vi "raster_scan_ground_shutter_new1.vi"() -> ()   [LabVIEW 2014] (continued)
  out "Spectra":cluster{"X":dbl, "Y":dbl}[](graph)=[{"X"=0.0, "Y"=0.9945769033962795}, {"X"=1.0, "Y"=0.9947742774918267}, {"X"=2.0, "Y"=0.9948669642938777}, {"X"=3.0, "Y"=0.9936503120864774}, {"X"=4.0, "Y"=0.99410258502573}, {"X"=5.0, "Y"=0.9940668724529786}, {"X"=6.0, "Y"=0.9937261199251147}, {"X"=7.0, "Y"=0.9931260471704962}, {"X"=8.0, "Y"=0.992983146361495}, {"X"=9.0, "Y"=0.9929502642830587}, {"X"=10.0, "Y"=0.993348571521516}, {"X"=11.0, "Y"=0.993598876753815}, {"X"=12.0, "Y"=0.9934939146853311}, {"X"=13.0, "Y"=0.994586396575504}, {"X"=14.0, "Y"=0.9948678392216669}, {"X"=15.0, "Y"=0.9949446767024206}, {"X"=16.0, "Y"=0.9954073186324625}, {"X"=17.0, "Y"=0.9946994697141236}, {"X"=18.0, "Y"=0.9944550521013112}, {"X"=19.0, "Y"=0.9944548626426379}, {"X"=20.0, "Y"=0.9935020518216698}, {"X"=21.0, "Y"=0.993658626270429}, {"X"=22.0, "Y"=0.9930985706701053}, {"X"=23.0, "Y"=0.9927409549288653}, {"X"=24.0, "Y"=0.9933271800562766}, {"X"=25.0, "Y"=0.9933239327867504}, {"X"=26.0, "Y"=0.9936027818310011}, {"X"=27.0, "Y"=0.9941736390892316}, {"X"=28.0, "Y"=0.9944683191284457}, {"X"=29.0, "Y"=0.9946912128001987}, {"X"=30.0, "Y"=0.9949701648247575}, {"X"=31.0, "Y"=0.9954933893926244}, {"X"=32.0, "Y"=0.9953930559005679}, {"X"=33.0, "Y"=0.9953512482962834}, {"X"=34.0, "Y"=0.9949945889014346}, {"X"=35.0, "Y"=0.9945846796005057}, {"X"=36.0, "Y"=0.9945806119423862}, {"X"=37.0, "Y"=0.9940680651637547}, {"X"=38.0, "Y"=0.9934632136375385}, {"X"=39.0, "Y"=0.9938541294612084}, {"X"=40.0, "Y"=0.9939211970775383}, {"X"=41.0, "Y"=0.9943574368554471}, {"X"=42.0, "Y"=0.9940101330545833}, {"X"=43.0, "Y"=0.9951367236173629}, {"X"=44.0, "Y"=0.9947572071731021}, {"X"=45.0, "Y"=0.9959756804722151}, {"X"=46.0, "Y"=0.9956182213866881}, {"X"=47.0, "Y"=0.9955081448310908}, {"X"=48.0, "Y"=0.995631614186444}, {"X"=49.0, "Y"=0.9956208296036213}, {"X"=50.0, "Y"=0.9962532896605993}, {"X"=51.0, "Y"=0.9962533556114832}, {"X"=52.0, "Y"=0.9958614347766488}, {"X"=53.0, "Y"=0.9957461636865907}, {"X"=54.0, "Y"=0.9956406167835943}, {"X"=55.0, "Y"=0.9956854770758357}, {"X"=56.0, "Y"=0.9956615767212665}, {"X"=57.0, "Y"=0.9956945496935939}, {"X"=58.0, "Y"=0.9962324646454884}, {"X"=59.0, "Y"=0.9964947407469643}, {"X"=60.0, "Y"=0.9970926126529994}, {"X"=61.0, "Y"=0.9968670550577037}, {"X"=62.0, "Y"=0.9970965802345466}, {"X"=63.0, "Y"=0.9972656492697479}, {"X"=64.0, "Y"=0.9968582713175153}, {"X"=65.0, "Y"=0.9970401597074343}, {"X"=66.0, "Y"=0.9970443003613348}, {"X"=67.0, "Y"=0.9973501158902985}, {"X"=68.0, "Y"=0.9981303427188236}, {"X"=69.0, "Y"=0.9977305631322807}, {"X"=70.0, "Y"=0.9977540022221576}, {"X"=71.0, "Y"=0.9979177515384777}, {"X"=72.0, "Y"=0.9977070175561394}, {"X"=73.0, "Y"=0.9982594221394903}, {"X"=74.0, "Y"=0.9980605550971688}, {"X"=75.0, "Y"=0.9978803843894963}, {"X"=76.0, "Y"=0.9980351530513635}, {"X"=77.0, "Y"=0.997851075793747}, {"X"=78.0, "Y"=0.9977894200446173}, {"X"=79.0, "Y"=0.9980636064837063}, {"X"=80.0, "Y"=0.9985695417684551}, {"X"=81.0, "Y"=0.9983812791956344}, {"X"=82.0, "Y"=0.998341559725945}, {"X"=83.0, "Y"=0.9986510426559164}, {"X"=84.0, "Y"=0.9991944690408153}, {"X"=85.0, "Y"=0.9995105354611745}, {"X"=86.0, "Y"=0.9991164177012709}, {"X"=87.0, "Y"=0.9995787032972646}, {"X"=88.0, "Y"=0.999454788017559}, {"X"=89.0, "Y"=0.999155685132651}, {"X"=90.0, "Y"=0.9987649485431911}, {"X"=91.0, "Y"=0.9986068010093291}, {"X"=92.0, "Y"=0.9976290609707013}, {"X"=93.0, "Y"=0.9981984662044825}, {"X"=94.0, "Y"=0.9977038350208027}, {"X"=95.0, "Y"=0.9979091185166017}, {"X"=96.0, "Y"=0.9984387389872107}, {"X"=97.0, "Y"=0.998465208764674}, {"X"=98.0, "Y"=0.9984988692668328}, {"X"=99.0, "Y"=0.9985777685951757}, {"X"=100.0, "Y"=0.9992981103342568}, {"X"=101.0, "Y"=0.9992176789240342}, {"X"=102.0, "Y"=0.9993160506202576}, {"X"=103.0, "Y"=0.9989016439374092}, {"X"=104.0, "Y"=0.998344902827914}, {"X"=105.0, "Y"=0.9982534949398687}, {"X"=106.0, "Y"=0.9981679578327937}, {"X"=107.0, "Y"=0.9971053281612066}, {"X"=108.0, "Y"=0.9971389132184889}, {"X"=109.0, "Y"=0.9963932015726795}, {"X"=110.0, "Y"=0.997024447798127}, {"X"=111.0, "Y"=0.9970324424009313}, {"X"=112.0, "Y"=0.9965660403857277}, {"X"=113.0, "Y"=0.9967183745842016}, {"X"=114.0, "Y"=0.9964512134239439}, {"X"=115.0, "Y"=0.9970165326649953}, {"X"=116.0, "Y"=0.9970951875378874}, {"X"=117.0, "Y"=0.9973005892418015}, {"X"=118.0, "Y"=0.9963413510352245}, {"X"=119.0, "Y"=0.9971948818360715}, {"X"=120.0, "Y"=0.9965308996775175}, {"X"=121.0, "Y"=0.9963267133794433}, {"X"=122.0, "Y"=0.9962490289924059}, {"X"=123.0, "Y"=0.99548039025524}, {"X"=124.0, "Y"=0.9948693730639996}, {"X"=125.0, "Y"=0.9944480660225795}, {"X"=126.0, "Y"=0.9946001681176279}, {"X"=127.0, "Y"=0.9943400299459262}, {"X"=128.0, "Y"=0.9946766752271496}, {"X"=129.0, "Y"=0.9950541253232607}, {"X"=130.0, "Y"=0.9945720808080813}, {"X"=131.0, "Y"=0.9948365747834916}, {"X"=132.0, "Y"=0.9950096816408889}, {"X"=133.0, "Y"=0.9949251864213772}, {"X"=134.0, "Y"=0.9940405960933386}, {"X"=135.0, "Y"=0.9938257461507851}, {"X"=136.0, "Y"=0.9944341634194976}, {"X"=137.0, "Y"=0.9940765135946166}, {"X"=138.0, "Y"=0.9932345009989546}, {"X"=139.0, "Y"=0.9928583382361931}, {"X"=140.0, "Y"=0.9926401294064278}, {"X"=141.0, "Y"=0.9929389318614823}, {"X"=142.0, "Y"=0.9927168132710366}, {"X"=143.0, "Y"=0.9926980851100657}, {"X"=144.0, "Y"=0.9920478801636552}, {"X"=145.0, "Y"=0.9925539606832021}, {"X"=146.0, "Y"=0.9928183067524887}, {"X"=147.0, "Y"=0.9926309997007406}, {"X"=148.0, "Y"=0.9917379549723951}, {"X"=149.0, "Y"=0.9923930264472043}, {"X"=150.0, "Y"=0.9918422229407143}, {"X"=151.0, "Y"=0.9914120672419391}, {"X"=152.0, "Y"=0.99163739825362}, {"X"=153.0, "Y"=0.9919110399406977}, {"X"=154.0, "Y"=0.9921509491520646}, {"X"=155.0, "Y"=0.9919826244448052}, {"X"=156.0, "Y"=0.9915638810734073}, {"X"=157.0, "Y"=0.9919883739976783}, {"X"=158.0, "Y"=0.9920186750240084}, {"X"=159.0, "Y"=0.9919484618380446}, {"X"=160.0, "Y"=0.9914327944146301}, {"X"=161.0, "Y"=0.9914833838660724}, {"X"=162.0, "Y"=0.9909328552617234}, {"X"=163.0, "Y"=0.99087425566013}, {"X"=164.0, "Y"=0.9896353008053395}, {"X"=165.0, "Y"=0.9901551379155719}, {"X"=166.0, "Y"=0.9892554727011702}, {"X"=167.0, "Y"=0.9900682622175773}, {"X"=168.0, "Y"=0.9897916508753934}, {"X"=169.0, "Y"=0.990067512842968}, {"X"=170.0, "Y"=0.9899459386432332}, {"X"=171.0, "Y"=0.9911563889695773}, {"X"=172.0, "Y"=0.9906125677236967}, {"X"=173.0, "Y"=0.9911465853056776}, {"X"=174.0, "Y"=0.9909635003778303}, {"X"=175.0, "Y"=0.9904879603894554}, {"X"=176.0, "Y"=0.9906311459060286}, {"X"=177.0, "Y"=0.9901740860080628}, {"X"=178.0, "Y"=0.9897736777248581}, {"X"=179.0, "Y"=0.9891083590917772}, {"X"=180.0, "Y"=0.9885407356391681}, {"X"=181.0, "Y"=0.9887437574853996}, {"X"=182.0, "Y"=0.9875871706582002}, {"X"=183.0, "Y"=0.9884301915828902}, {"X"=184.0, "Y"=0.9880786140088792}, {"X"=185.0, "Y"=0.9888277232763419}, {"X"=186.0, "Y"=0.9890520421386713}, {"X"=187.0, "Y"=0.9895665359857829}, {"X"=188.0, "Y"=0.9899055459783636}, {"X"=189.0, "Y"=0.9904301218378724}, {"X"=190.0, "Y"=0.9902234343017942}, {"X"=191.0, "Y"=0.9901724736185524}, {"X"=192.0, "Y"=0.9901434464237711}, {"X"=193.0, "Y"=0.9895637959186443}, {"X"=194.0, "Y"=0.988702010117804}, {"X"=195.0, "Y"=0.9881102735335884}, {"X"=196.0, "Y"=0.9876271197301395}, {"X"=197.0, "Y"=0.9870059351949232}, {"X"=198.0, "Y"=0.987547568608782}, {"X"=199.0, "Y"=0.9873805981457269}, {"X"=200.0, "Y"=0.9876423646840112}, {"X"=201.0, "Y"=0.9881306949826341}, {"X"=202.0, "Y"=0.9878880960676789}, {"X"=203.0, "Y"=0.9892054326780412}, {"X"=204.0, "Y"=0.9883302594497589}, {"X"=205.0, "Y"=0.9893826274122949}, {"X"=206.0, "Y"=0.9892849007020629}, {"X"=207.0, "Y"=0.9890527115412554}, {"X"=208.0, "Y"=0.9889256316402685}, {"X"=209.0, "Y"=0.9887361369286901}, {"X"=210.0, "Y"=0.9878797445751826}, {"X"=211.0, "Y"=0.9877112444891087}, {"X"=212.0, "Y"=0.9877868727003994}, {"X"=213.0, "Y"=0.9874769504690166}, {"X"=214.0, "Y"=0.9871655257657367}, {"X"=215.0, "Y"=0.9871507163512597}, {"X"=216.0, "Y"=0.987264000932457}, {"X"=217.0, "Y"=0.9872537012488534}, {"X"=218.0, "Y"=0.9878563327045027}, {"X"=219.0, "Y"=0.9879033062040963}, {"X"=220.0, "Y"=0.9882991906907304}, {"X"=221.0, "Y"=0.9887480998872463}, {"X"=222.0, "Y"=0.9881367601151576}, {"X"=223.0, "Y"=0.9880177726421817}, {"X"=224.0, "Y"=0.9883156195990628}, {"X"=225.0, "Y"=0.9879355258074888}, {"X"=226.0, "Y"=0.9880262146308868}, {"X"=227.0, "Y"=0.9878205873870225}, {"X"=228.0, "Y"=0.9879979695910659}, {"X"=229.0, "Y"=0.9875604094133309}, {"X"=230.0, "Y"=0.9873140506915336}, {"X"=231.0, "Y"=0.9877819716694046}, {"X"=232.0, "Y"=0.9871561041420477}, {"X"=233.0, "Y"=0.9879116486306354}, {"X"=234.0, "Y"=0.9886438705239039}, {"X"=235.0, "Y"=0.9882990214645868}, {"X"=236.0, "Y"=0.9879251504436052}, {"X"=237.0, "Y"=0.9885682799078236}, {"X"=238.0, "Y"=0.9882975691220256}, {"X"=239.0, "Y"=0.98809140019495}, {"X"=240.0, "Y"=0.9872249435387722}, {"X"=241.0, "Y"=0.9874254589398946}, {"X"=242.0, "Y"=0.9883584962911233}, {"X"=243.0, "Y"=0.9877210265121739}, {"X"=244.0, "Y"=0.9889044731576114}, {"X"=245.0, "Y"=0.9889998621680584}, {"X"=246.0, "Y"=0.9887562610924129}, {"X"=247.0, "Y"=0.9889233646870126}, {"X"=248.0, "Y"=0.9886205539813097}, {"X"=249.0, "Y"=0.9889017231973711}, {"X"=250.0, "Y"=0.9892196969470405}, {"X"=251.0, "Y"=0.9892281944234239}, {"X"=252.0, "Y"=0.9888604304511662}, {"X"=253.0, "Y"=0.9890505246826924}, {"X"=254.0, "Y"=0.9890154370177213}, {"X"=255.0, "Y"=0.9891772241501933}, {"X"=256.0, "Y"=0.988832118915806}, {"X"=257.0, "Y"=0.9886118021975259}, {"X"=258.0, "Y"=0.9889802132148718}, {"X"=259.0, "Y"=0.9892806336265826}, {"X"=260.0, "Y"=0.9895329690616291}, {"X"=261.0, "Y"=0.9904042662027042}, {"X"=262.0, "Y"=0.9908231520975864}, {"X"=263.0, "Y"=0.9909121720252757}, {"X"=264.0, "Y"=0.9913133878792242}, {"X"=265.0, "Y"=0.9911264642288832}, {"X"=266.0, "Y"=0.9907064200980509}, {"X"=267.0, "Y"=0.9907593652845151}, {"X"=268.0, "Y"=0.9907705633561275}, {"X"=269.0, "Y"=0.9904878226282635}, {"X"=270.0, "Y"=0.9908187861127447}, {"X"=271.0, "Y"=0.9906254696326791}, {"X"=272.0, "Y"=0.9905573181977684}, {"X"=273.0, "Y"=0.9905800885486153}, {"X"=274.0, "Y"=0.9912109420696134}, {"X"=275.0, "Y"=0.9914824697505557}, {"X"=276.0, "Y"=0.992227115706744}, {"X"=277.0, "Y"=0.99285414389668}, {"X"=278.0, "Y"=0.9927929387816049}, {"X"=279.0, "Y"=0.9933197570768701}, {"X"=280.0, "Y"=0.9934331338352567}, {"X"=281.0, "Y"=0.9934008840881473}, {"X"=282.0, "Y"=0.9935287240841545}, {"X"=283.0, "Y"=0.9938253031705743}, {"X"=284.0, "Y"=0.993498601147894}, {"X"=285.0, "Y"=0.9935112494120911}, {"X"=286.0, "Y"=0.9932030351865082}, {"X"=287.0, "Y"=0.9935321643793682}, {"X"=288.0, "Y"=0.9935338962125877}, {"X"=289.0, "Y"=0.9940572304924011}, {"X"=290.0, "Y"=0.9939962423550712}, {"X"=291.0, "Y"=0.9940039939894947}, {"X"=292.0, "Y"=0.9951419214649302}, {"X"=293.0, "Y"=0.9958152481189801}, {"X"=294.0, "Y"=0.9956744187967643}, {"X"=295.0, "Y"=0.9957859054898696}, {"X"=296.0, "Y"=0.9963597432442338}, {"X"=297.0, "Y"=0.9963464806444049}, {"X"=298.0, "Y"=0.996565547598631}, {"X"=299.0, "Y"=0.9970456149544855}, {"X"=300.0, "Y"=0.9962488669230711}, {"X"=301.0, "Y"=0.9964034672765409}, {"X"=302.0, "Y"=0.9962665778829146}, {"X"=303.0, "Y"=0.9962049855918085}, {"X"=304.0, "Y"=0.9968841226218517}, {"X"=305.0, "Y"=0.9966428477570376}, {"X"=306.0, "Y"=0.9972464803560432}, {"X"=307.0, "Y"=0.9967008713434102}, {"X"=308.0, "Y"=0.9976084960484286}, {"X"=309.0, "Y"=0.9975185002731412}, {"X"=310.0, "Y"=0.9983983890371154}, {"X"=311.0, "Y"=0.9982974444908385}, {"X"=312.0, "Y"=0.9987052789761125}, {"X"=313.0, "Y"=0.9982691360022389}, {"X"=314.0, "Y"=0.9987512050963647}, {"X"=315.0, "Y"=0.9982950838816262}, {"X"=316.0, "Y"=0.9982986815469811}, {"X"=317.0, "Y"=0.9989451067310545}, {"X"=318.0, "Y"=0.9994812319476775}, {"X"=319.0, "Y"=0.9987637602173738}, {"X"=320.0, "Y"=0.9986816151807595}, {"X"=321.0, "Y"=0.9990808249950823}, {"X"=322.0, "Y"=0.9992449023297956}, {"X"=323.0, "Y"=0.999275153648}, {"X"=324.0, "Y"=1.0003732573061601}, {"X"=325.0, "Y"=0.9991965310240539}, {"X"=326.0, "Y"=0.999569233917549}, {"X"=327.0, "Y"=1.0005284020049339}, {"X"=328.0, "Y"=1.0004096588220222}, {"X"=329.0, "Y"=1.0003846709577688}, {"X"=330.0, "Y"=1.000270884798537}, {"X"=331.0, "Y"=1.0001374636437872}, {"X"=332.0, "Y"=1.0001594575787047}, {"X"=333.0, "Y"=1.0001761506267028}, {"X"=334.0, "Y"=1.000165247299422}, {"X"=335.0, "Y"=1.0004438418020443}, {"X"=336.0, "Y"=1.0004078128172427}, {"X"=337.0, "Y"=1.000141608271659}, {"X"=338.0, "Y"=0.9999310798724922}, {"X"=339.0, "Y"=1.0000051443789508}, {"X"=340.0, "Y"=1.000258051791045}, {"X"=341.0, "Y"=1.0007536458809314}, {"X"=342.0, "Y"=1.0003656545944697}, {"X"=343.0, "Y"=1.0004163295116526}, {"X"=344.0, "Y"=1.0004724212647915}, {"X"=345.0, "Y"=1.0004967058476173}, {"X"=346.0, "Y"=0.9999857278586478}, {"X"=347.0, "Y"=0.9998290175235972}, {"X"=348.0, "Y"=0.9999327038090732}, {"X"=349.0, "Y"=1.000209077856183}, {"X"=350.0, "Y"=0.9999334642825315}, {"X"=351.0, "Y"=1.0002194807373026}, {"X"=352.0, "Y"=1.0001609447323363}, {"X"=353.0, "Y"=1.0005675012269715}, {"X"=354.0, "Y"=0.9999348034932509}, {"X"=355.0, "Y"=0.9998910417937119}, {"X"=356.0, "Y"=0.9992376163758537}, {"X"=357.0, "Y"=1.000229604088896}, {"X"=358.0, "Y"=0.9996110087834967}, {"X"=359.0, "Y"=0.9996709480973932}, {"X"=360.0, "Y"=0.9993900541132547}, {"X"=361.0, "Y"=0.9994399097419068}, {"X"=362.0, "Y"=0.9989804444753528}, {"X"=363.0, "Y"=0.9988148494816306}, {"X"=364.0, "Y"=0.9986814697104245}, {"X"=365.0, "Y"=0.9989859590100776}, {"X"=366.0, "Y"=0.9989630194348239}, {"X"=367.0, "Y"=0.9986929061238093}, {"X"=368.0, "Y"=0.999368246512584}, {"X"=369.0, "Y"=0.9993397157764048}, {"X"=370.0, "Y"=0.9992161295804917}, {"X"=371.0, "Y"=0.9996741200878309}, {"X"=372.0, "Y"=0.9987958090783459}, {"X"=373.0, "Y"=0.9986220017821499}, {"X"=374.0, "Y"=0.9983827589387424}, {"X"=375.0, "Y"=0.9986217425320943}, {"X"=376.0, "Y"=0.9988276526224658}, {"X"=377.0, "Y"=0.9983371715200989}, {"X"=378.0, "Y"=0.9978993937962697}, {"X"=379.0, "Y"=0.997519976021216}, {"X"=380.0, "Y"=0.9974571313883922}, {"X"=381.0, "Y"=0.9978694341745249}, {"X"=382.0, "Y"=0.9969600723549592}, {"X"=383.0, "Y"=0.9978975540996382}, {"X"=384.0, "Y"=0.9975797315910041}, {"X"=385.0, "Y"=0.9980891705188358}, {"X"=386.0, "Y"=0.9976623784178721}, {"X"=387.0, "Y"=0.9974094268186124}, {"X"=388.0, "Y"=0.9976285075136032}, {"X"=389.0, "Y"=0.9972604747410225}, {"X"=390.0, "Y"=0.9969852894175658}, {"X"=391.0, "Y"=0.9971986944330739}, {"X"=392.0, "Y"=0.9967703633191467}, {"X"=393.0, "Y"=0.9969739032416945}, {"X"=394.0, "Y"=0.9963516797770992}, {"X"=395.0, "Y"=0.9969924397437879}, {"X"=396.0, "Y"=0.9966974642266633}, {"X"=397.0, "Y"=0.9965202826092788}, {"X"=398.0, "Y"=0.9957110058508749}, {"X"=399.0, "Y"=0.9963166472992203}, {"X"=400.0, "Y"=0.9965632873842588}, {"X"=401.0, "Y"=0.9964199433569914}, {"X"=402.0, "Y"=0.9966838817491888}, {"X"=403.0, "Y"=0.9972472774524763}, {"X"=404.0, "Y"=0.9961702127759391}, {"X"=405.0, "Y"=0.9963391248405309}, {"X"=406.0, "Y"=0.9959628235351379}, {"X"=407.0, "Y"=0.9958302300724778}, {"X"=408.0, "Y"=0.9961046814276435}, {"X"=409.0, "Y"=0.9961486233956509}, {"X"=410.0, "Y"=0.9959642564254102}, {"X"=411.0, "Y"=0.9960013843813469}, {"X"=412.0, "Y"=0.9953815457888371}, {"X"=413.0, "Y"=0.9959366649291765}, {"X"=414.0, "Y"=0.9963551144568551}, {"X"=415.0, "Y"=0.9953598205062505}, {"X"=416.0, "Y"=0.9953001805913673}, {"X"=417.0, "Y"=0.9954990354706129}, {"X"=418.0, "Y"=0.9959610609749414}, {"X"=419.0, "Y"=0.9956888805818223}, {"X"=420.0, "Y"=0.9960947787394934}, {"X"=421.0, "Y"=0.9958175145335946}, {"X"=422.0, "Y"=0.9954639723611227}, {"X"=423.0, "Y"=0.9950560259849376}, {"X"=424.0, "Y"=0.9951304465212562}, {"X"=425.0, "Y"=0.9958458986290973}, {"X"=426.0, "Y"=0.9953648899549052}, {"X"=427.0, "Y"=0.9950754626127001}, {"X"=428.0, "Y"=0.9952492454136798}, {"X"=429.0, "Y"=0.99523013530319}, {"X"=430.0, "Y"=0.9945859201123685}, {"X"=431.0, "Y"=0.9950245730198668}, {"X"=432.0, "Y"=0.9955208628359311}, {"X"=433.0, "Y"=0.9947991988066446}, {"X"=434.0, "Y"=0.9955691055942305}, {"X"=435.0, "Y"=0.9950343442079201}, {"X"=436.0, "Y"=0.9951984441413309}, {"X"=437.0, "Y"=0.9954773057676222}, {"X"=438.0, "Y"=0.9951800972435834}, {"X"=439.0, "Y"=0.9951219608087896}, {"X"=440.0, "Y"=0.9952438849998119}, {"X"=441.0, "Y"=0.9943483979721591}, {"X"=442.0, "Y"=0.995174387512307}, {"X"=443.0, "Y"=0.9950486986680683}, {"X"=444.0, "Y"=0.9952920758720216}, {"X"=445.0, "Y"=0.9952343756356732}, {"X"=446.0, "Y"=0.9953573574172749}, {"X"=447.0, "Y"=0.994887176531457}, {"X"=448.0, "Y"=0.9956901536251682}, {"X"=449.0, "Y"=0.9953081676288387}, {"X"=450.0, "Y"=0.9956306739275201}, {"X"=451.0, "Y"=0.9952047513921564}, {"X"=452.0, "Y"=0.9951094940049702}, {"X"=453.0, "Y"=0.9955580359473676}, {"X"=454.0, "Y"=0.9957000003590071}, {"X"=455.0, "Y"=0.9959349261252317}, {"X"=456.0, "Y"=0.9951675787972696}, {"X"=457.0, "Y"=0.9952534864653381}, {"X"=458.0, "Y"=0.9947675908555841}, {"X"=459.0, "Y"=0.9952255756881186}, {"X"=460.0, "Y"=0.9955999597225985}, {"X"=461.0, "Y"=0.9957210809601894}, {"X"=462.0, "Y"=0.9962219187126349}, {"X"=463.0, "Y"=0.9950253118473475}, {"X"=464.0, "Y"=0.9952746511661845}, {"X"=465.0, "Y"=0.9955955039410045}, {"X"=466.0, "Y"=0.9953537198652035}, {"X"=467.0, "Y"=0.9957253897668253}, {"X"=468.0, "Y"=0.9953236482233332}, {"X"=469.0, "Y"=0.9953822156108794}, {"X"=470.0, "Y"=0.9958591038091335}, {"X"=471.0, "Y"=0.9957506257501119}, {"X"=472.0, "Y"=0.9955790409849812}, {"X"=473.0, "Y"=0.9953090658693439}, {"X"=474.0, "Y"=0.9947915478095556}, {"X"=475.0, "Y"=0.9954268300450004}, {"X"=476.0, "Y"=0.995262677167648}, {"X"=477.0, "Y"=0.9954973282349253}, {"X"=478.0, "Y"=0.9955090001050857}, {"X"=479.0, "Y"=0.9960544790358801}, {"X"=480.0, "Y"=0.9956670470710183}, {"X"=481.0, "Y"=0.9958933961556072}, {"X"=482.0, "Y"=0.996345076269324}, {"X"=483.0, "Y"=0.9961327862202871}, {"X"=484.0, "Y"=0.9961666748004979}, {"X"=485.0, "Y"=0.9958929183577934}, {"X"=486.0, "Y"=0.9960499891424248}, {"X"=487.0, "Y"=0.9955770807979752}, {"X"=488.0, "Y"=0.9957331364463746}, {"X"=489.0, "Y"=0.9952766318019293}, {"X"=490.0, "Y"=0.9956181131678156}, {"X"=491.0, "Y"=0.9952386179240643}, {"X"=492.0, "Y"=0.9957556804360669}, {"X"=493.0, "Y"=0.995792130851567}, {"X"=494.0, "Y"=0.9956885845493915}, {"X"=495.0, "Y"=0.9958446919182999}, {"X"=496.0, "Y"=0.9958074557545651}, {"X"=497.0, "Y"=0.9964205123451934}, {"X"=498.0, "Y"=0.9965256657513467}, {"X"=499.0, "Y"=0.9959730784207221}, {"X"=500.0, "Y"=0.9963841460143855}, {"X"=501.0, "Y"=0.9961407997731256}, {"X"=502.0, "Y"=0.9963119080015646}, {"X"=503.0, "Y"=0.9967965671005882}, {"X"=504.0, "Y"=0.9963653097240543}, {"X"=505.0, "Y"=0.9963783983392102}, {"X"=506.0, "Y"=0.9961759742592253}, {"X"=507.0, "Y"=0.9966982563472333}, {"X"=508.0, "Y"=0.9960776777111763}, {"X"=509.0, "Y"=0.9957480951942244}, {"X"=510.0, "Y"=0.9964484006101223}, {"X"=511.0, "Y"=0.9963066807096024}, {"X"=512.0, "Y"=0.9962390429931123}, {"X"=513.0, "Y"=0.9966745858122457}, {"X"=514.0, "Y"=0.9968898487353313}, {"X"=515.0, "Y"=0.9970603478626283}, {"X"=516.0, "Y"=0.9970412520555734}, {"X"=517.0, "Y"=0.9974441543069041}, {"X"=518.0, "Y"=0.9975296723108728}, {"X"=519.0, "Y"=0.997630677970172}, {"X"=520.0, "Y"=0.9976035050729387}, {"X"=521.0, "Y"=0.9967475021044707}, {"X"=522.0, "Y"=0.9974703810459983}, {"X"=523.0, "Y"=0.9973304831802989}, {"X"=524.0, "Y"=0.9967303837490574}, {"X"=525.0, "Y"=0.996863485783012}, {"X"=526.0, "Y"=0.9969179220536531}, {"X"=527.0, "Y"=0.9969108680284032}, {"X"=528.0, "Y"=0.9971759118498723}, {"X"=529.0, "Y"=0.9973803539652828}, {"X"=530.0, "Y"=0.9971381720463038}, {"X"=531.0, "Y"=0.997976023644964}, {"X"=532.0, "Y"=0.997748764676727}, {"X"=533.0, "Y"=0.9979042869155424}, {"X"=534.0, "Y"=0.9979757589489487}, {"X"=535.0, "Y"=0.9974718594056934}, {"X"=536.0, "Y"=0.9977082494542683}, {"X"=537.0, "Y"=0.9979039956689645}, {"X"=538.0, "Y"=0.9973644111432559}, {"X"=539.0, "Y"=0.9979110028346743}, {"X"=540.0, "Y"=0.9977147369742246}, {"X"=541.0, "Y"=0.9982517409612547}, {"X"=542.0, "Y"=0.9974188824432151}, {"X"=543.0, "Y"=0.9977654877175895}, {"X"=544.0, "Y"=0.9978545183540273}, {"X"=545.0, "Y"=0.9978954802718253}, {"X"=546.0, "Y"=0.9978847126029841}, {"X"=547.0, "Y"=0.9986282274099947}, {"X"=548.0, "Y"=0.9985592746779094}, {"X"=549.0, "Y"=0.9984101644173519}, {"X"=550.0, "Y"=0.9981985424776665}, {"X"=551.0, "Y"=0.998426104497088}, {"X"=552.0, "Y"=0.9985691286987668}, {"X"=553.0, "Y"=0.9979689171383916}, {"X"=554.0, "Y"=0.9982460987713048}, {"X"=555.0, "Y"=0.998121473974186}, {"X"=556.0, "Y"=0.9977379675030132}, {"X"=557.0, "Y"=0.998243375619955}, {"X"=558.0, "Y"=0.998132359067814}, {"X"=559.0, "Y"=0.9983256230790136}, {"X"=560.0, "Y"=0.9980172261705131}, {"X"=561.0, "Y"=0.9984771190185349}, {"X"=562.0, "Y"=0.9979225481535584}, {"X"=563.0, "Y"=0.9981209325830508}, {"X"=564.0, "Y"=0.9981205014531911}, {"X"=565.0, "Y"=0.9985116348563284}, {"X"=566.0, "Y"=0.9985313300015474}, {"X"=567.0, "Y"=0.9985618507511264}, {"X"=568.0, "Y"=0.9980731056228417}, {"X"=569.0, "Y"=0.99777584834941}, {"X"=570.0, "Y"=0.9983204895779979}, {"X"=571.0, "Y"=0.9979093460943547}, {"X"=572.0, "Y"=0.9974202665539573}, {"X"=573.0, "Y"=0.9974138091852186}, {"X"=574.0, "Y"=0.99811669466617}, {"X"=575.0, "Y"=0.9981038738953151}, {"X"=576.0, "Y"=0.9977082372079878}, {"X"=577.0, "Y"=0.9980030461884963}, {"X"=578.0, "Y"=0.9980034114768427}, {"X"=579.0, "Y"=0.9982364510217848}, {"X"=580.0, "Y"=0.9979325576022529}, {"X"=581.0, "Y"=0.9977734094940269}, {"X"=582.0, "Y"=0.9981140314943433}, {"X"=583.0, "Y"=0.9979539107254143}, {"X"=584.0, "Y"=0.997655931871743}, {"X"=585.0, "Y"=0.9972543054374033}, {"X"=586.0, "Y"=0.9969317121833642}, {"X"=587.0, "Y"=0.9968443093625065}, {"X"=588.0, "Y"=0.9966413383535035}, {"X"=589.0, "Y"=0.9960249116592703}, {"X"=590.0, "Y"=0.9963089300738579}, {"X"=591.0, "Y"=0.9961840817664352}, {"X"=592.0, "Y"=0.9963553748195709}, {"X"=593.0, "Y"=0.9962705798119079}, {"X"=594.0, "Y"=0.99670571106408}, {"X"=595.0, "Y"=0.9964327341637447}, {"X"=596.0, "Y"=0.9965823060297267}, {"X"=597.0, "Y"=0.9968535449226337}, {"X"=598.0, "Y"=0.9965539588406062}, {"X"=599.0, "Y"=0.9961449417496469}, {"X"=600.0, "Y"=0.9965984047900572}, {"X"=601.0, "Y"=0.9962586900884038}, {"X"=602.0, "Y"=0.9962103374424071}, {"X"=603.0, "Y"=0.9954906975090069}, {"X"=604.0, "Y"=0.9957365549620107}, {"X"=605.0, "Y"=0.9963388156166715}, {"X"=606.0, "Y"=0.9965861993129}, {"X"=607.0, "Y"=0.9974232683784019}, {"X"=608.0, "Y"=0.9992020432658635}, {"X"=609.0, "Y"=1.00039405639493}, {"X"=610.0, "Y"=1.0013783401587335}, {"X"=611.0, "Y"=1.0033275791215845}, {"X"=612.0, "Y"=1.0047939581934993}, {"X"=613.0, "Y"=1.0072483446876968}, {"X"=614.0, "Y"=1.008871757151934}, {"X"=615.0, "Y"=1.0110282901417909}, {"X"=616.0, "Y"=1.013371337166815}, {"X"=617.0, "Y"=1.0151009747430668}, {"X"=618.0, "Y"=1.0176425122069255}, {"X"=619.0, "Y"=1.0197495431887913}, {"X"=620.0, "Y"=1.0224688407170561}, {"X"=621.0, "Y"=1.0247490900420204}, {"X"=622.0, "Y"=1.0276990459376787}, {"X"=623.0, "Y"=1.0296095041094517}, {"X"=624.0, "Y"=1.0333078315506532}, {"X"=625.0, "Y"=1.0362685626177792}, {"X"=626.0, "Y"=1.038924641533091}, {"X"=627.0, "Y"=1.041572265389145}, {"X"=628.0, "Y"=1.0435587138867348}, {"X"=629.0, "Y"=1.0464705907166}, {"X"=630.0, "Y"=1.0490032103492144}, {"X"=631.0, "Y"=1.050504978522211}, {"X"=632.0, "Y"=1.0528251069017325}, {"X"=633.0, "Y"=1.0534239144824968}, {"X"=634.0, "Y"=1.0549006626365562}, {"X"=635.0, "Y"=1.0550592680988555}, {"X"=636.0, "Y"=1.0549458189191194}, {"X"=637.0, "Y"=1.0549779342343906}, {"X"=638.0, "Y"=1.0539315349680067}, {"X"=639.0, "Y"=1.0542361563716711}, {"X"=640.0, "Y"=1.0534478719509481}, {"X"=641.0, "Y"=1.052399132550848}, {"X"=642.0, "Y"=1.0514082647686147}, {"X"=643.0, "Y"=1.0504137881143336}, {"X"=644.0, "Y"=1.0488047450457352}, {"X"=645.0, "Y"=1.0477270368509513}, {"X"=646.0, "Y"=1.045690156385211}, {"X"=647.0, "Y"=1.0432872265980713}, {"X"=648.0, "Y"=1.0410317960687832}, {"X"=649.0, "Y"=1.0379447532276453}, {"X"=650.0, "Y"=1.0348336539420064}, {"X"=651.0, "Y"=1.0315576847668324}, {"X"=652.0, "Y"=1.028862670120101}, {"X"=653.0, "Y"=1.0258567044055389}, {"X"=654.0, "Y"=1.0230131849598842}, {"X"=655.0, "Y"=1.0209637506857185}, {"X"=656.0, "Y"=1.0181556258277114}, {"X"=657.0, "Y"=1.0160814779436314}, {"X"=658.0, "Y"=1.0136796020817032}, {"X"=659.0, "Y"=1.0120789147322529}, {"X"=660.0, "Y"=1.0104539182883303}, {"X"=661.0, "Y"=1.008677968134813}, {"X"=662.0, "Y"=1.0068674140821063}, {"X"=663.0, "Y"=1.005416554572116}, {"X"=664.0, "Y"=1.004418287860281}, {"X"=665.0, "Y"=1.0026019255081793}, {"X"=666.0, "Y"=1.001755051681397}, {"X"=667.0, "Y"=1.0007427244836384}, {"X"=668.0, "Y"=1.000212255121392}, {"X"=669.0, "Y"=1.0001516680923108}, {"X"=670.0, "Y"=1.0002951868519772}, {"X"=671.0, "Y"=0.9997153062030121}, {"X"=672.0, "Y"=0.9996816416219783}, {"X"=673.0, "Y"=0.9998761682577347}, {"X"=674.0, "Y"=0.9992615693650128}, {"X"=675.0, "Y"=1.000324398030068}, {"X"=676.0, "Y"=0.9999570200209895}, {"X"=677.0, "Y"=1.0000117210295363}, {"X"=678.0, "Y"=1.0000634134316824}, {"X"=679.0, "Y"=1.0001331522973944}, {"X"=680.0, "Y"=1.0004081949275365}, {"X"=681.0, "Y"=0.9998829901655063}, {"X"=682.0, "Y"=1.000187544558325}, {"X"=683.0, "Y"=1.0003801314997531}, {"X"=684.0, "Y"=1.0003149177046684}, {"X"=685.0, "Y"=0.9998517079056821}, {"X"=686.0, "Y"=1.0004100893131052}, {"X"=687.0, "Y"=1.0000016158957639}, {"X"=688.0, "Y"=1.0006017898810222}, {"X"=689.0, "Y"=1.0005718409574569}, {"X"=690.0, "Y"=1.0007007698411632}, {"X"=691.0, "Y"=1.000506938601441}, {"X"=692.0, "Y"=1.0000772828380353}, {"X"=693.0, "Y"=1.0005686668319205}, {"X"=694.0, "Y"=1.0009164301763613}, {"X"=695.0, "Y"=1.0004825673685438}, {"X"=696.0, "Y"=1.000543465394958}, {"X"=697.0, "Y"=1.00084754089509}, {"X"=698.0, "Y"=1.0006573921442272}, {"X"=699.0, "Y"=1.0008281174083582}, {"X"=700.0, "Y"=1.001000500464312}, {"X"=701.0, "Y"=1.0005876920760894}, {"X"=702.0, "Y"=1.000993095286034}, {"X"=703.0, "Y"=1.00056708158604}, {"X"=704.0, "Y"=1.0006259107721924}, {"X"=705.0, "Y"=1.0007697612854025}, {"X"=706.0, "Y"=1.000978106387117}, {"X"=707.0, "Y"=1.0007664078085046}, {"X"=708.0, "Y"=1.0011454626210547}, {"X"=709.0, "Y"=1.0011091615448482}, {"X"=710.0, "Y"=1.001056081943534}, {"X"=711.0, "Y"=1.0012334014028355}, {"X"=712.0, "Y"=1.0011837250778726}, {"X"=713.0, "Y"=1.000916622339644}, {"X"=714.0, "Y"=1.0012569862720535}, {"X"=715.0, "Y"=1.0009918254170156}, {"X"=716.0, "Y"=1.0007201726153137}, {"X"=717.0, "Y"=1.0011288843771156}, {"X"=718.0, "Y"=1.0008681092115939}, {"X"=719.0, "Y"=1.0009798044664915}, {"X"=720.0, "Y"=1.001112027329558}, {"X"=721.0, "Y"=1.0010204159387182}, {"X"=722.0, "Y"=1.0006192087669428}, {"X"=723.0, "Y"=1.0012939973290147}, {"X"=724.0, "Y"=1.0007005394153075}, {"X"=725.0, "Y"=1.0009357538518868}, {"X"=726.0, "Y"=1.0014740988896245}, {"X"=727.0, "Y"=1.0010121967650842}, {"X"=728.0, "Y"=1.0016954160298988}, {"X"=729.0, "Y"=1.0011144874969538}, {"X"=730.0, "Y"=1.000975865976058}, {"X"=731.0, "Y"=1.0011789828226225}, {"X"=732.0, "Y"=1.0011893085482935}, {"X"=733.0, "Y"=1.0011614230048504}, {"X"=734.0, "Y"=1.0011976845828305}, {"X"=735.0, "Y"=1.0011581305715418}, {"X"=736.0, "Y"=1.0010556075044197}, {"X"=737.0, "Y"=1.000937577300871}, {"X"=738.0, "Y"=1.0009325997585012}, {"X"=739.0, "Y"=1.0007734996223567}, {"X"=740.0, "Y"=1.0008682847275774}, {"X"=741.0, "Y"=1.0009267272013356}, {"X"=742.0, "Y"=1.0009202446313439}, {"X"=743.0, "Y"=1.0011286199467828}, {"X"=744.0, "Y"=1.0009420307972523}, {"X"=745.0, "Y"=1.0011039647090711}, {"X"=746.0, "Y"=1.0009233724169802}, {"X"=747.0, "Y"=1.0007503724260123}, {"X"=748.0, "Y"=1.0008308485115536}, {"X"=749.0, "Y"=1.0009287533631965}, {"X"=750.0, "Y"=1.0007719252489964}, {"X"=751.0, "Y"=1.0008692070915899}, {"X"=752.0, "Y"=1.0008582123092458}, {"X"=753.0, "Y"=1.0005798712787062}, {"X"=754.0, "Y"=1.0009749912624057}, {"X"=755.0, "Y"=1.0009132421180837}, {"X"=756.0, "Y"=1.0006067695791088}, {"X"=757.0, "Y"=1.0006890331168343}, {"X"=758.0, "Y"=1.0008962054677861}, {"X"=759.0, "Y"=1.0005844554606693}, {"X"=760.0, "Y"=1.0008238897141335}, {"X"=761.0, "Y"=1.0008713716200581}, {"X"=762.0, "Y"=1.000462698368419}, {"X"=763.0, "Y"=1.00038551560003}, {"X"=764.0, "Y"=1.0005740364073854}, {"X"=765.0, "Y"=1.0010253429662304}, {"X"=766.0, "Y"=1.0003632657418395}, {"X"=767.0, "Y"=1.000567308693705}, {"X"=768.0, "Y"=1.000286790348577}, {"X"=769.0, "Y"=1.0004665761914815}, {"X"=770.0, "Y"=1.000168483840905}, {"X"=771.0, "Y"=1.000152637463018}, {"X"=772.0, "Y"=1.000214242192368}, {"X"=773.0, "Y"=1.0003869867588742}, {"X"=774.0, "Y"=1.0005376955714191}, {"X"=775.0, "Y"=1.0004800558745468}, {"X"=776.0, "Y"=1.0005707911790136}, {"X"=777.0, "Y"=0.9997487173368662}, {"X"=778.0, "Y"=1.0004505353589024}, {"X"=779.0, "Y"=1.0006358048732418}, {"X"=780.0, "Y"=1.0006913500666466}, {"X"=781.0, "Y"=1.0000594857246996}, {"X"=782.0, "Y"=1.000202033665066}, {"X"=783.0, "Y"=1.0005896258602271}, {"X"=784.0, "Y"=0.9998116953891122}, {"X"=785.0, "Y"=1.0000030368836728}, {"X"=786.0, "Y"=0.9999692468282858}, {"X"=787.0, "Y"=0.9996749236190133}, {"X"=788.0, "Y"=0.9999528813725637}, {"X"=789.0, "Y"=0.9996934968232128}, {"X"=790.0, "Y"=1.0001246386179192}, {"X"=791.0, "Y"=1.000121231707337}, {"X"=792.0, "Y"=1.0003574387962126}, {"X"=793.0, "Y"=0.9998897647562817}, {"X"=794.0, "Y"=0.999991814875864}, {"X"=795.0, "Y"=0.9999717796372998}, {"X"=796.0, "Y"=0.9999164248339153}, {"X"=797.0, "Y"=1.0000472803501612}, {"X"=798.0, "Y"=1.0003096307675872}, {"X"=799.0, "Y"=0.9995521439215307}, {"X"=800.0, "Y"=0.9998268441921865}, {"X"=801.0, "Y"=0.9997823002205563}, {"X"=802.0, "Y"=0.9997914401002861}, {"X"=803.0, "Y"=0.999436665219622}, {"X"=804.0, "Y"=0.9996389638963711}, {"X"=805.0, "Y"=0.999683035386018}, {"X"=806.0, "Y"=0.9999043749665063}, {"X"=807.0, "Y"=0.999872375868445}, {"X"=808.0, "Y"=0.9995564412851898}, {"X"=809.0, "Y"=0.9997146784363528}, {"X"=810.0, "Y"=0.9992468990944221}, {"X"=811.0, "Y"=0.9999100681507468}, {"X"=812.0, "Y"=0.9996803844051546}, {"X"=813.0, "Y"=0.999812736922049}, {"X"=814.0, "Y"=0.9999079641000937}, {"X"=815.0, "Y"=0.9995712757348625}, {"X"=816.0, "Y"=0.9999753952150852}, {"X"=817.0, "Y"=0.9996161230527898}, {"X"=818.0, "Y"=0.9999692827506793}, {"X"=819.0, "Y"=0.9997854374958309}, {"X"=820.0, "Y"=0.9997379623488489}, {"X"=821.0, "Y"=0.9997951408693897}, {"X"=822.0, "Y"=0.9996005558855302}, {"X"=823.0, "Y"=0.9996013042279536}, {"X"=824.0, "Y"=0.9994527699487141}, {"X"=825.0, "Y"=0.9994611971332913}, {"X"=826.0, "Y"=0.9995943046267404}, {"X"=827.0, "Y"=0.9993996315141247}, {"X"=828.0, "Y"=0.999466764473007}, {"X"=829.0, "Y"=0.9997275186993784}, {"X"=830.0, "Y"=0.9994655220422562}, {"X"=831.0, "Y"=0.9999217304306618}, {"X"=832.0, "Y"=0.9995485361962716}, {"X"=833.0, "Y"=0.9998723066127978}, {"X"=834.0, "Y"=0.9995042794915885}, {"X"=835.0, "Y"=0.9995245056820103}, {"X"=836.0, "Y"=0.9991550561955388}, {"X"=837.0, "Y"=0.9996330482905573}, {"X"=838.0, "Y"=0.9999634602317182}, {"X"=839.0, "Y"=0.999554498145934}, {"X"=840.0, "Y"=0.9993969166206773}, {"X"=841.0, "Y"=0.9994570922088231}, {"X"=842.0, "Y"=0.9994160747857141}, {"X"=843.0, "Y"=0.9995563480657043}, {"X"=844.0, "Y"=0.9999575192332566}, {"X"=845.0, "Y"=0.9994287267946973}, {"X"=846.0, "Y"=0.9997828708624986}, {"X"=847.0, "Y"=0.9997294658304303}, {"X"=848.0, "Y"=0.9997987491676308}, {"X"=849.0, "Y"=0.9998366805189256}, {"X"=850.0, "Y"=0.9998421980321909}, {"X"=851.0, "Y"=0.9997708290381001}, {"X"=852.0, "Y"=0.9997571893188337}, {"X"=853.0, "Y"=0.9999425601459052}, {"X"=854.0, "Y"=0.999591626867619}, {"X"=855.0, "Y"=0.9997575945123861}, {"X"=856.0, "Y"=0.9998259214523023}, {"X"=857.0, "Y"=0.9998524142922023}, {"X"=858.0, "Y"=0.9998214349671982}, {"X"=859.0, "Y"=0.9996982431382163}, {"X"=860.0, "Y"=1.000006724215444}, {"X"=861.0, "Y"=0.9997226946982664}, {"X"=862.0, "Y"=1.0001222798385383}, {"X"=863.0, "Y"=0.9997723680899672}, {"X"=864.0, "Y"=1.0004691521323734}, {"X"=865.0, "Y"=0.9995317329722564}, {"X"=866.0, "Y"=0.9999706638370606}, {"X"=867.0, "Y"=0.9999485081385426}, {"X"=868.0, "Y"=1.0002513015681866}, {"X"=869.0, "Y"=1.0001094834288995}, {"X"=870.0, "Y"=1.0000796165289747}, {"X"=871.0, "Y"=1.0001052236277999}, {"X"=872.0, "Y"=1.0004937362292834}, {"X"=873.0, "Y"=1.000013590642817}, {"X"=874.0, "Y"=1.0003573287643348}, {"X"=875.0, "Y"=1.0004525481711148}, {"X"=876.0, "Y"=0.9999755900094128}, {"X"=877.0, "Y"=1.0003964124631561}, {"X"=878.0, "Y"=1.0005363708541122}, {"X"=879.0, "Y"=1.0004557806466459}, {"X"=880.0, "Y"=1.000733510349076}, {"X"=881.0, "Y"=1.0002652087127946}, {"X"=882.0, "Y"=1.0003971179645745}, {"X"=883.0, "Y"=1.0006048161778602}, {"X"=884.0, "Y"=1.0005937878882152}, {"X"=885.0, "Y"=1.000476561139529}, {"X"=886.0, "Y"=1.0004827953448545}, {"X"=887.0, "Y"=1.000421392196533}, {"X"=888.0, "Y"=1.0003776494746428}, {"X"=889.0, "Y"=1.0002335494105024}, {"X"=890.0, "Y"=1.0005818770177213}, {"X"=891.0, "Y"=1.000556169743754}, {"X"=892.0, "Y"=1.0005142471348096}, {"X"=893.0, "Y"=1.0006009804720526}, {"X"=894.0, "Y"=1.000462567319067}, {"X"=895.0, "Y"=1.0004232511191642}, {"X"=896.0, "Y"=1.0002985391510821}, {"X"=897.0, "Y"=1.000563080763287}, {"X"=898.0, "Y"=1.0003985868488332}, {"X"=899.0, "Y"=1.0005921693519613}, {"X"=900.0, "Y"=1.0005517113896354}, {"X"=901.0, "Y"=1.0004511874507864}, {"X"=902.0, "Y"=1.0003164509105338}, {"X"=903.0, "Y"=1.0006514699992903}, {"X"=904.0, "Y"=1.0004630517353699}, {"X"=905.0, "Y"=1.0003696899849848}, {"X"=906.0, "Y"=1.0000750343598261}, {"X"=907.0, "Y"=1.0001652803283667}, {"X"=908.0, "Y"=1.0005821961595347}, {"X"=909.0, "Y"=1.0000753056610996}, {"X"=910.0, "Y"=1.0008381429666606}, {"X"=911.0, "Y"=1.0002009630275162}, {"X"=912.0, "Y"=1.0000090046202812}, {"X"=913.0, "Y"=1.000357217161673}, {"X"=914.0, "Y"=1.0005551947210591}, {"X"=915.0, "Y"=1.0006019344688362}, {"X"=916.0, "Y"=1.0003157102839864}, {"X"=917.0, "Y"=1.0006539638821532}, {"X"=918.0, "Y"=1.0004523550286122}, {"X"=919.0, "Y"=1.0004362081948674}, {"X"=920.0, "Y"=1.0004658381122902}, {"X"=921.0, "Y"=1.0005032431132526}, {"X"=922.0, "Y"=1.0006496135004674}, {"X"=923.0, "Y"=1.000421409515476}, {"X"=924.0, "Y"=1.00029741571484}, {"X"=925.0, "Y"=1.0003752604308016}, {"X"=926.0, "Y"=1.0000674401177483}, {"X"=927.0, "Y"=1.000752504898771}, {"X"=928.0, "Y"=1.0004265589119117}, {"X"=929.0, "Y"=1.000277485793791}, {"X"=930.0, "Y"=1.000143732812286}, {"X"=931.0, "Y"=1.000586072623539}, {"X"=932.0, "Y"=1.0003218460655414}, {"X"=933.0, "Y"=1.000253779745408}, {"X"=934.0, "Y"=0.9999684895073191}, {"X"=935.0, "Y"=1.0000553542910315}, {"X"=936.0, "Y"=1.0004387435193063}, {"X"=937.0, "Y"=1.0005796043709154}, {"X"=938.0, "Y"=1.0002239035981928}, {"X"=939.0, "Y"=1.0005100497007755}, {"X"=940.0, "Y"=1.000276926115426}, {"X"=941.0, "Y"=1.0005393916224292}, {"X"=942.0, "Y"=1.0003102290640964}, {"X"=943.0, "Y"=1.0004510828201474}, {"X"=944.0, "Y"=1.0004024270555596}, {"X"=945.0, "Y"=1.0003071722234138}, {"X"=946.0, "Y"=1.0003479438286045}, {"X"=947.0, "Y"=1.0006054265939661}, {"X"=948.0, "Y"=1.0004341205130898}, {"X"=949.0, "Y"=1.0005543120812839}, {"X"=950.0, "Y"=1.0004009168011205}, {"X"=951.0, "Y"=1.0006692411711766}, {"X"=952.0, "Y"=1.0005684966442148}, {"X"=953.0, "Y"=1.0002059600051625}, {"X"=954.0, "Y"=1.0004913192089357}, {"X"=955.0, "Y"=1.0003185704962576}, {"X"=956.0, "Y"=1.0003571139773684}, {"X"=957.0, "Y"=1.0004792329148344}, {"X"=958.0, "Y"=1.0007107646312456}, {"X"=959.0, "Y"=1.0003472703541094}, {"X"=960.0, "Y"=1.00055060436529}, {"X"=961.0, "Y"=1.0002969671654476}, {"X"=962.0, "Y"=1.0002867873822994}, {"X"=963.0, "Y"=1.0003786420047431}, {"X"=964.0, "Y"=1.0003682377805028}, {"X"=965.0, "Y"=1.0005896761650959}, {"X"=966.0, "Y"=1.0003457782727248}, {"X"=967.0, "Y"=1.0006909634949526}, {"X"=968.0, "Y"=1.0001113405044946}, {"X"=969.0, "Y"=1.0003299278640605}, {"X"=970.0, "Y"=1.0006022370584085}, {"X"=971.0, "Y"=1.0002903312662772}, {"X"=972.0, "Y"=1.0005061770542671}, {"X"=973.0, "Y"=1.0004220088897762}, {"X"=974.0, "Y"=1.00062971722216}, {"X"=975.0, "Y"=1.0003765492341081}, {"X"=976.0, "Y"=1.0004592871043285}, {"X"=977.0, "Y"=1.000514847516494}, {"X"=978.0, "Y"=1.0003467113971076}, {"X"=979.0, "Y"=1.0002069450901978}, {"X"=980.0, "Y"=1.0005040498159148}, {"X"=981.0, "Y"=1.000138336954979}, {"X"=982.0, "Y"=1.000390235537673}, {"X"=983.0, "Y"=1.000504818092738}, {"X"=984.0, "Y"=1.0002436968618853}, {"X"=985.0, "Y"=1.0004223209898575}, {"X"=986.0, "Y"=1.0002155513016582}, {"X"=987.0, "Y"=1.0001190993872675}, {"X"=988.0, "Y"=1.000394310225494}, {"X"=989.0, "Y"=1.0004553646966243}, {"X"=990.0, "Y"=1.0001042595318252}, {"X"=991.0, "Y"=1.000235823625573}, {"X"=992.0, "Y"=1.0002616383711564}, {"X"=993.0, "Y"=1.0003022919280078}, {"X"=994.0, "Y"=1.000557447133573}, {"X"=995.0, "Y"=1.0002431232712843}, {"X"=996.0, "Y"=1.000407779249664}, {"X"=997.0, "Y"=1.0001910030091277}, {"X"=998.0, "Y"=1.0000811448918354}, {"X"=999.0, "Y"=1.000409690537901}, {"X"=1000.0, "Y"=1.0003398218940822}, {"X"=1001.0, "Y"=1.000204245610935}, {"X"=1002.0, "Y"=1.00018533413993}, {"X"=1003.0, "Y"=1.000302314225904}, {"X"=1004.0, "Y"=1.0002923742421739}, {"X"=1005.0, "Y"=1.000309364574194}, {"X"=1006.0, "Y"=1.0000426923874066}, {"X"=1007.0, "Y"=1.0004618206725626}, {"X"=1008.0, "Y"=1.0003141108219815}, {"X"=1009.0, "Y"=1.0005023576969727}, {"X"=1010.0, "Y"=1.0003544772082134}, {"X"=1011.0, "Y"=1.0004524090568325}, {"X"=1012.0, "Y"=1.0001465182625013}, {"X"=1013.0, "Y"=1.0002729209887085}, {"X"=1014.0, "Y"=1.0003807048184004}, {"X"=1015.0, "Y"=1.0000934145436753}, {"X"=1016.0, "Y"=1.000523744822201}, {"X"=1017.0, "Y"=1.0003810050685418}, {"X"=1018.0, "Y"=1.0001897441615633}, {"X"=1019.0, "Y"=1.0000433790093919}, {"X"=1020.0, "Y"=1.0002344668735443}, {"X"=1021.0, "Y"=1.0000743430369654}, {"X"=1022.0, "Y"=1.0005123321725913}, {"X"=1023.0, "Y"=0.9999867984833275}, {"X"=1024.0, "Y"=1.00028886416398}, {"X"=1025.0, "Y"=0.9999976564025252}, {"X"=1026.0, "Y"=1.000147489191159}, {"X"=1027.0, "Y"=1.0001021283303542}, {"X"=1028.0, "Y"=1.0004207742794315}, {"X"=1029.0, "Y"=1.0003511315237172}, {"X"=1030.0, "Y"=1.0002740488978419}, {"X"=1031.0, "Y"=1.0005715604928058}, {"X"=1032.0, "Y"=1.0000849731377497}, {"X"=1033.0, "Y"=1.000664325326948}, {"X"=1034.0, "Y"=1.0002715158858457}, {"X"=1035.0, "Y"=1.0004068426842052}, {"X"=1036.0, "Y"=1.0003341226908409}, {"X"=1037.0, "Y"=1.0003845014598438}, {"X"=1038.0, "Y"=1.000382059982626}, {"X"=1039.0, "Y"=1.0002566925098917}, {"X"=1040.0, "Y"=1.0004394237268197}, {"X"=1041.0, "Y"=1.0003796791309603}, {"X"=1042.0, "Y"=1.0005573908410998}, {"X"=1043.0, "Y"=1.0003274420534478}, {"X"=1044.0, "Y"=1.000649864733999}, {"X"=1045.0, "Y"=1.0001894757842382}, {"X"=1046.0, "Y"=1.0003630377518922}, {"X"=1047.0, "Y"=1.0007311125223617}, {"X"=1048.0, "Y"=1.0003937967302898}, {"X"=1049.0, "Y"=1.0004660000627263}, {"X"=1050.0, "Y"=1.000370743171769}, {"X"=1051.0, "Y"=1.0003895018697897}, {"X"=1052.0, "Y"=1.0003660457840664}, {"X"=1053.0, "Y"=1.0006618337709967}, {"X"=1054.0, "Y"=1.0004746367542625}, {"X"=1055.0, "Y"=1.0006470220462966}, {"X"=1056.0, "Y"=1.000336358127014}, {"X"=1057.0, "Y"=1.0004776161543254}, {"X"=1058.0, "Y"=1.0005350625396425}, {"X"=1059.0, "Y"=1.0007114086431932}, {"X"=1060.0, "Y"=1.0005461150814388}, {"X"=1061.0, "Y"=1.0001568330212558}, {"X"=1062.0, "Y"=1.0006049675270903}, {"X"=1063.0, "Y"=1.0008072532845746}, {"X"=1064.0, "Y"=1.0007899340972959}, {"X"=1065.0, "Y"=1.0003705264800233}, {"X"=1066.0, "Y"=1.000663501831443}, {"X"=1067.0, "Y"=1.0003968148498383}, {"X"=1068.0, "Y"=1.0004410295865593}, {"X"=1069.0, "Y"=1.000990825072581}, {"X"=1070.0, "Y"=1.0007069226291818}, {"X"=1071.0, "Y"=1.0009074944245333}, {"X"=1072.0, "Y"=1.000986596814561}, {"X"=1073.0, "Y"=1.0006469461319005}, {"X"=1074.0, "Y"=1.0006961161864978}, {"X"=1075.0, "Y"=1.0009206991231543}, {"X"=1076.0, "Y"=1.0004970130469557}, {"X"=1077.0, "Y"=1.0008897415638358}, {"X"=1078.0, "Y"=1.0004689157169488}, {"X"=1079.0, "Y"=1.0008271789537952}, {"X"=1080.0, "Y"=1.0005958642457493}, {"X"=1081.0, "Y"=1.0006627201543532}, {"X"=1082.0, "Y"=1.000911669123488}, {"X"=1083.0, "Y"=1.0007669752129835}, {"X"=1084.0, "Y"=1.0007869594284737}, 
